vi "ReduceRowsTDMS.vi"(5 "Max Rows":i32, 8 "error in":errorcluster, 10 "Array":string[][](array[string]), 11 "semaphore":T1) -> (0 "error out":errorcluster, 3 "semaphore out":T1)   [LabVIEW 2015]
panel:
  out "canal":string
  out "grupo":string
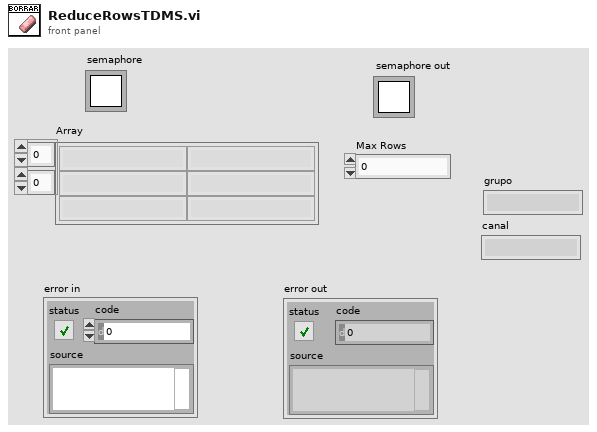
[diagram p1: front panel]
types:
  T1 = typedef "Semaphore RefNum" = refnum<k1>
  T2 = enum16{"open", "open or create", "create or replace", "create", "open (read-only)"}
  T3 = cluster{"tdms control out":refnum<k34>, "tdms historial out":refnum<k34>, "tdms sinc out":refnum<k34>}
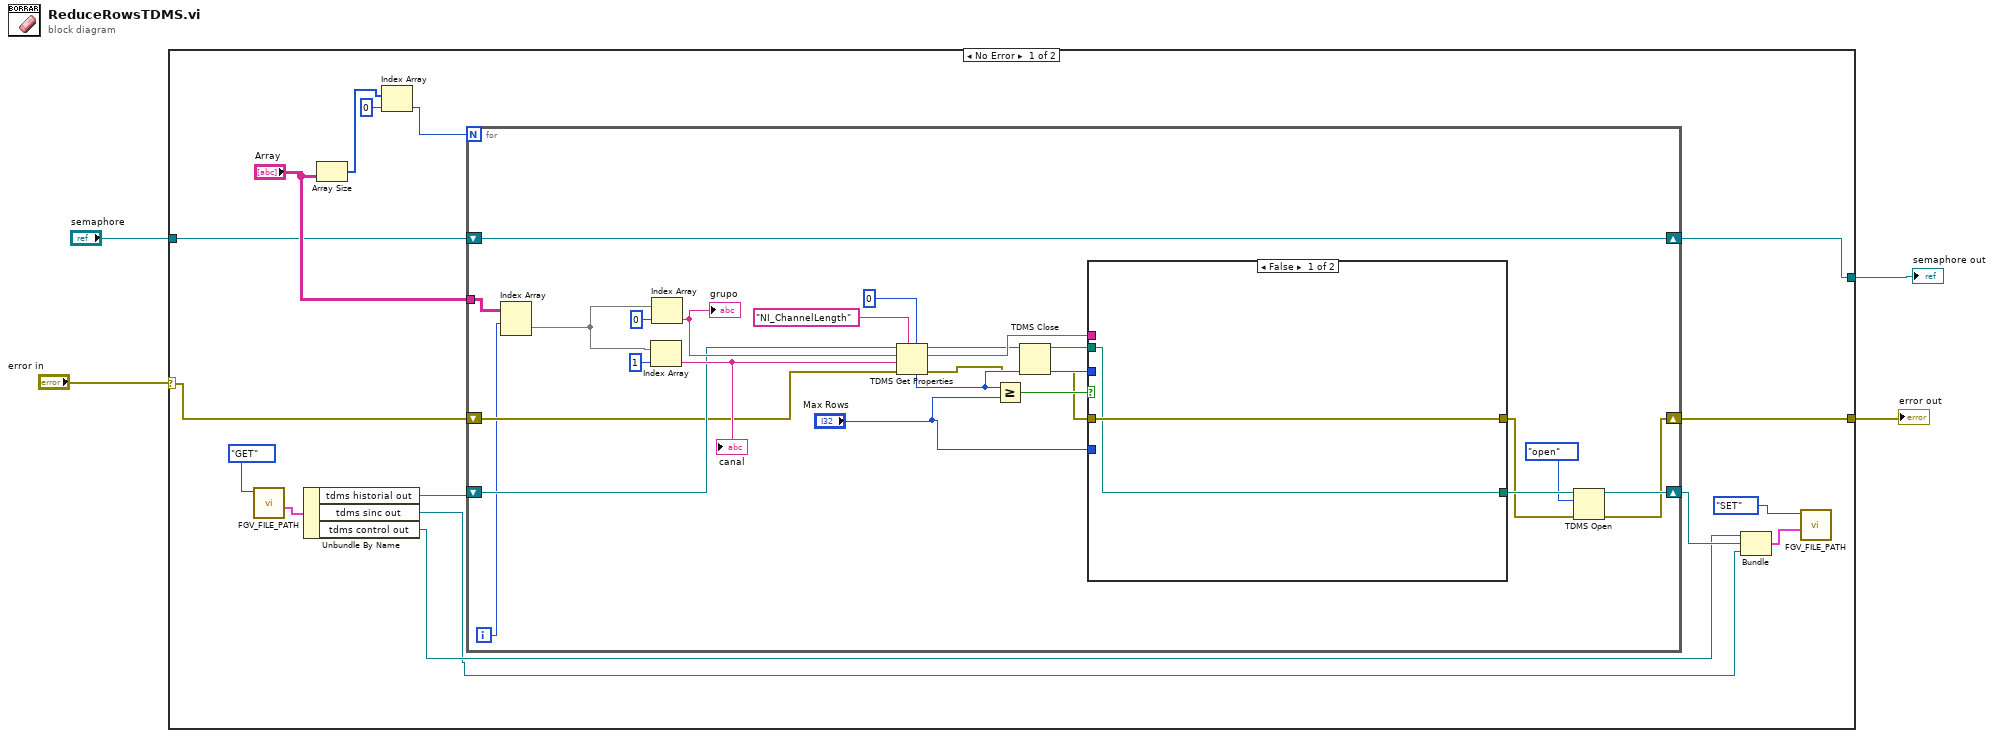
[diagram p0: block diagram]
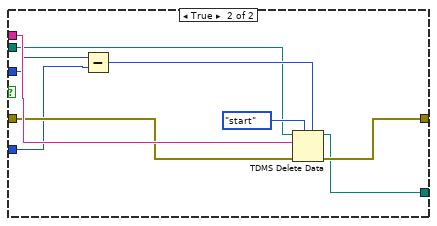
[diagram p2: hidden frame]
diagram:
  n1 = case shown="No Error" "error in" {
    selector: "error in" -> [w15 w58]
    tunnel: [w16 w58] -> w4
    tunnel: "semaphore" -> [w6 w57]
    tunnel: [w5 w57] -> w1
    frame No Error {
      n2 = call "FGV_FILE_PATH.vi"("Function"=enum16{"GET", "SET"}."GET") -> ("Data Out"=w8:T3)  [unwired: 10 in]
      n3 = Unbundle By Name(w8) -> ("tdms historial out"=w13:refnum<k34>, "tdms sinc out"=w10:refnum<k34>, "tdms control out"=w11:refnum<k34>)
      n4 = Array Size(array="Array") -> (size(s)=w20:i32[])
      n5 = Index Array(array=w20, index=0) -> (element=w18:i32)
      n6 = for {
        N: w18 -> [_]
        tunnel: "Array" -> [w23]
        shift-right: [w32] -> w12
        shift-left: w13 -> [w31]
        shift-right: [w28] -> w16
        shift-left: w15 -> [w30]
        shift-right: [w25] -> w5
        shift-left: w6 -> [w25]
        i -> [w21]
        n7 = Index Array(array=w23, index (row)=w21) -> (element=w22:string[])  [unwired: 1 in]
        n8 = Index Array(array=w22, index=1) -> (element=w34:string)
        "canal" <- w34
        n9 = Index Array(array=w22, index=0) -> (element=w36:string)
        "grupo" <- w36
        n10 = TDMS Get Properties(5:0, 7:"NI_ChannelLength" ("property name"), 8:w30, 9:w34, 10:w36, 11:w31) -> (0:w39:errorcluster, 2:w43:string, 3:w40:refnum<k34>, 4:w42:i32)  [unwired: 2 out]
        n11 = Greater Or Equal?(x=w42, y="Max Rows") -> (x >= y?=w44:bool)
        n12 = TDMS Close(8:w39, 11:w40) -> (0:w38:errorcluster, 3:w26:path)
        n13 = case shown="False" w44 {
          tunnel: w43 -> [_ w55]
          tunnel: w38 -> [w47 w54]
          tunnel: [w47 w53] -> w29
          tunnel: w42 -> [_ w52]
          tunnel: "Max Rows" -> [_ w51]
          tunnel: [w46 w49] -> w33
          tunnel: w26 -> [w46 w48]
          frame False {
          }
          frame True {
            n14 = Subtract(x=w52, y=w51) -> (x-y=w50:i32)
            n15 = TDMS Delete Data(5:w50, 7:enum16{"start", "end"}."start" ("from (0: start)"), 8:w54, 10:w55, 11:w48) -> (0:w53:errorcluster, 3:w49:path)  [unwired: 2 in]
          }
        }
        n16 = TDMS Open(8:w29, 10:T2."open" ("operation (0:open)"), 11:w33) -> (0:w28:errorcluster, 3:w32:refnum<k34>)  [unwired: 4 in]
      }
      n17 = Bundle("tdms control out"=w11, "tdms historial out"=w12, "tdms sinc out"=w10) -> (w9:T3)  [unwired: 1 in]
      n18 = call "FGV_FILE_PATH.vi"("Data In"=w9, "Function"=enum16{"GET", "SET"}."SET") -> ()  [unwired: 9 in, 1 out]
    }
    frame Error {
    }
  }
  "error out" <- w4
  "semaphore out" <- w1
